vi "uService GUI.vi"(8 "error in (no error)":errorcluster, 11 "Kasli Wrapper in":refnum<class "Kasli Wrapper 2.0.lvclass">=refnum) -> (3 "Kasli Wrapper out":refnum<class "Kasli Wrapper 2.0.lvclass">)   [LabVIEW 2020, in "CIRCUS_uServices.lvlib" / "Kasli Wrapper 2.0.lvlib" / "Kasli Wrapper 2.0.lvclass"]
uses:
  Kasli Wrapper 2.0.lvclass
  TALOS/TALOS_PPL.lvlibp/Father of all uServices/Father of all uServices/Father of all uServices.lvclass
  C:/Users/marco/Documents/GitHub_Lab/CIRCUS/TALOS/TALOS_PPL.lvlibp/Ancestor/Ancestor/Ancestor.lvclass
  C:/Users/marco/Documents/GitHub_Lab/CIRCUS/TALOS/Actor Framework.lvlibp/1abvi3w/vi.lib/ActorFramework/Actor/Actor.lvclass
  C:/Users/marco/Documents/GitHub_Lab/CIRCUS/TALOS/TALOS_PPL.lvlibp/Father of all uServices/Father of all uServices/Father of all uServices.lvclass
panel:
  out "RID":u32
  out "Kasli Configuration":string
  out "uS ID":string
  in  "Clear":bool
  out "Client StdErr":string
  out "Client StdOut":string
  out "ProcessExit":bool
  out "Master StdErr":string
  out "Master StdOut":string
  out "RUN!":bool
  in  "Script":string
  in  "Restart":bool
  in  "Submit Script":bool
  in  "stop New uService":bool
  in  "Init":bool
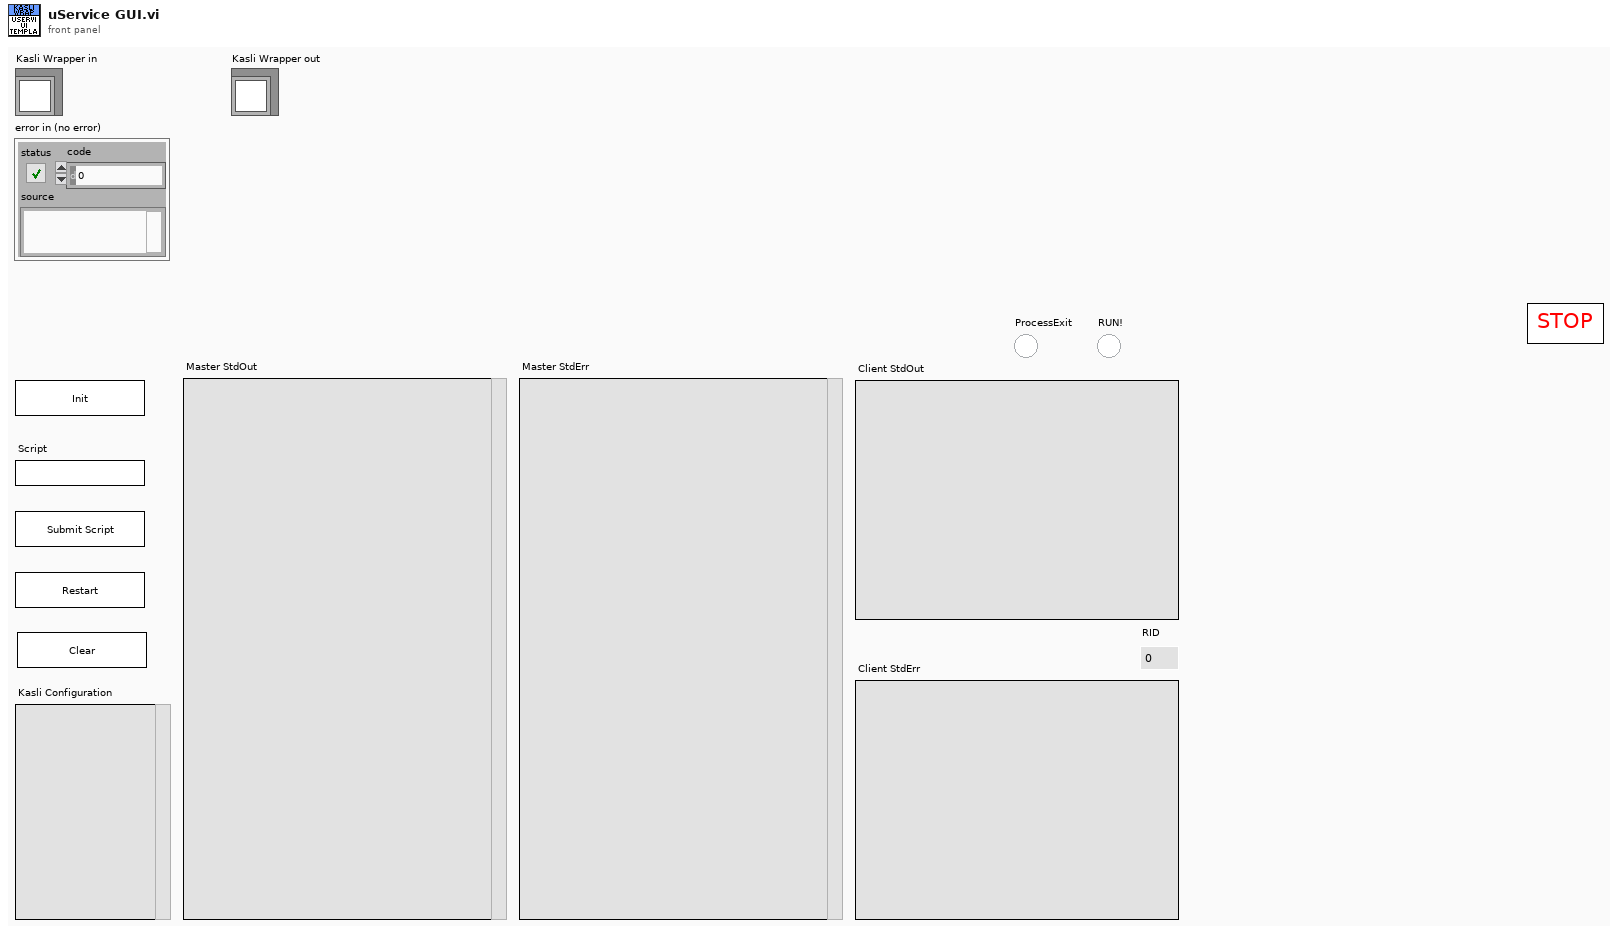
[diagram p1: front panel]
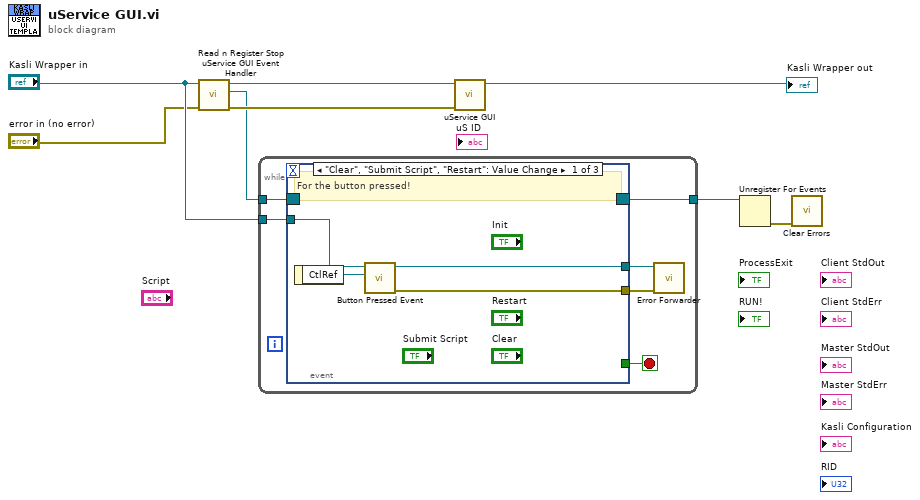
[diagram p0: block diagram]
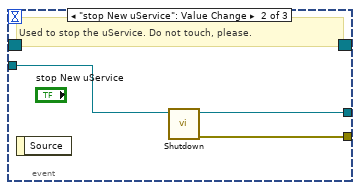
[diagram p2: hidden frame]
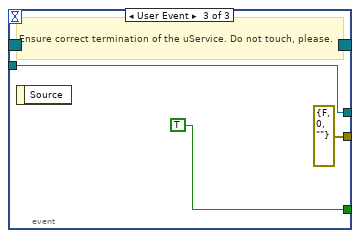
[diagram p3: hidden frame]
diagram:
  n1 = call-dynamic "Read n Register Stop uService GUI Event Handler .vi"("error in (no error)"="error in (no error)", "uService Template in"="Kasli Wrapper in") -> ("error out"=w6:errorcluster, "Stop uService GUI Event Ref"=w5:refnum<event-registration>, "uService Template out"=w7:refnum<class "Kasli Wrapper 2.0.lvclass">)  [unwired: 7 in]
  n2 = while {
    tunnel: [w14] -> w8
    tunnel: w5 -> [w12]
    tunnel: "Kasli Wrapper in" -> [w11]
    stop <- w13 stop-if-true
    n3 = event shown="[0] \"Clear\", \"Submit Script\", \"Restart\": Value Change" {
      selector: w12 -> [_ _ _]
      dyn-events: [_ _ _] -> w14
      timeout: _ -> [_ _ _]
      tunnel: [_ _ TRUE] -> w13
      tunnel: w11 -> [w18 w21 w23]
      tunnel: [w16 w20 w23] -> w10
      tunnel: [w15 w19 errorcluster {"status"=FALSE, "code"=0, "source"=""} ("error out")] -> w9
      event "Clear", "Submit Script", "Restart": Value Change {
        # "For the button pressed!"
        n4 = event-data() -> ("CtlRef"=w17:refnum<vi>)  [unwired: 1 in]
        n5 = call-dynamic "Button Pressed Event.vi"("CtlRef"=w17, "uService Template in"=w18) -> ("error out"=w15:errorcluster, "uService Template out"=w16:refnum<class "Kasli Wrapper 2.0.lvclass">)  [unwired: 8 in]
      }
      event "stop New uService": Value Change {
        # "Used to stop the uService. Do not touch, please."
        n6 = event-data() -> ()  [unwired: 1 in, 1 out]
        n7 = call "Shutdown.vi"("Father of all uServices in"=w21) -> ("error out"=w19:errorcluster, "Father of all uServices out"=w20:refnum<class "Father of all uServices.lvclass">)  [unwired: 9 in]
      }
      event User Event {
        # "Ensure correct termination of the uService. Do not touch, please."
        n8 = event-data() -> ()  [unwired: 1 in, 1 out]
      }
    }
    n9 = call "Error Forwarder.vi"("error in (no error)"=w9, "Father of all uServices in"=w10) -> ()  [unwired: 10 in]
  }
  n10 = call-parent "uService GUI.vi"("error in (no error)"=w6, "uService Template in"=w7) -> ("uService Template out"=→"Kasli Wrapper out":refnum<class "Kasli Wrapper 2.0.lvclass">)  [unwired: 9 in]
  n11 = Unregister For Events(event registration refnum=w8) -> (error out=w1:errorcluster)  [unwired: 1 in]
  n12 = call <vilib>:"Clear Errors.vi"("error in (no error)"=w1) -> ()  [unwired: 5 in, 2 out]
